vi "Actual PID Gyro.vi"(9 "Negate":bool=TRUE, 11 "Wanted End":dbl) -> (1 "Done":bool, 3 "Output":dbl)   [LabVIEW 2017]
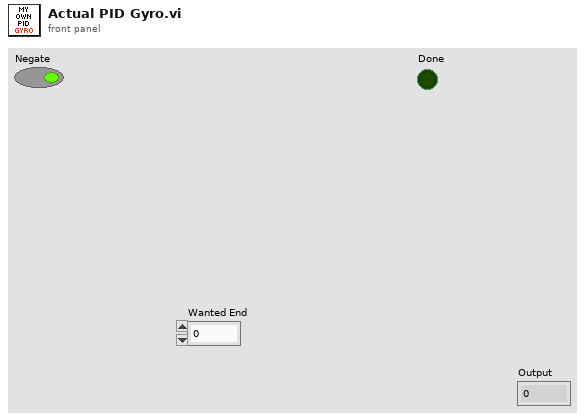
[diagram p1: front panel]
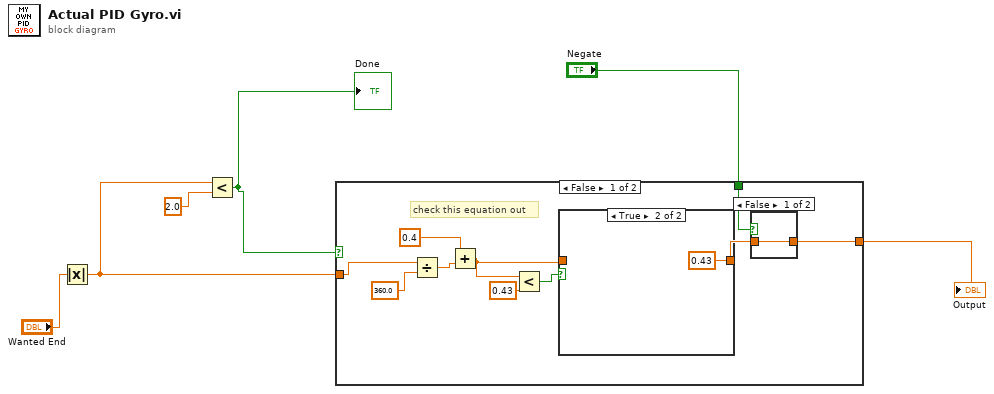
[diagram p0: block diagram]
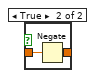
[diagram p2: hidden frame]
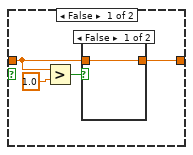
[diagram p3: hidden frame]
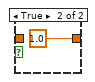
[diagram p4: hidden frame]
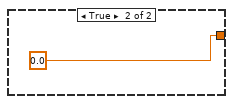
[diagram p5: hidden frame]
diagram:
  n1 = Absolute Value(x="Wanted End") -> (abs(x)=w1:dbl)
  n2 = Less?(x=w1, y=2.0) -> (x < y?=w2:bool)
  "Done" <- w2
  n3 = case shown="False" w2 {
    tunnel: "Negate" -> [w10 _]
    tunnel: [w8 0.0 ("y")] -> w3
    tunnel: w1 -> [w7 _]
    frame False {
      # "check this equation out"
      n4 = Divide(x=w7, y=360.0) -> (x/y=w15:dbl)
      n5 = Add(x=0.4 ("y"), y=w15) -> (x+y=w16:dbl)
      n6 = Less?(x=w16, y=0.43) -> (x < y?=w13:bool)
      n7 = case shown="True" w13 {
        tunnel: [w20 0.43 ("y")] -> w14
        tunnel: w16 -> [w21 _]
        frame False {
          n8 = Greater?(x=w21, y=1.0) -> (0:w23:bool)
          n9 = case shown="False" w23 {
            tunnel: w21 -> [w24 _]
            tunnel: [w24 1.0 ("y")] -> w20
            frame False {
            }
            frame True {
            }
          }
        }
        frame True {
        }
      }
      n10 = case shown="False" w10 {
        tunnel: w14 -> [w17 w19]
        tunnel: [w17 w18] -> w8
        frame False {
        }
        frame True {
          n11 = Negate(x=w19) -> (-x=w18:dbl)
        }
      }
    }
    frame True {
    }
  }
  "Output" <- w3
